vi "Get Device Type.vi"(8 "error in (no error)":errorcluster, 10 "config file refnum in":T2, 11 "IED in":refnum<class "IED.lvclass">) -> (0 "error out":errorcluster, 2 "config file refnum out":T2, 3 "IED out":refnum<class "IED.lvclass">, 4 "Device Type":T1)   [LabVIEW 2015, in "IED Actor.lvlib" / "IED.lvclass"]
uses:
  IED.lvclass
  <vilib>/Utility/config.llb/Config Data RefNum.ctl
  Controls/Device Type Enum.ctl
  <vilib>/Utility/config.llb/Read Key (String).vi
  <vilib>/Utility/config.llb/NI_LVConfig.lvlib
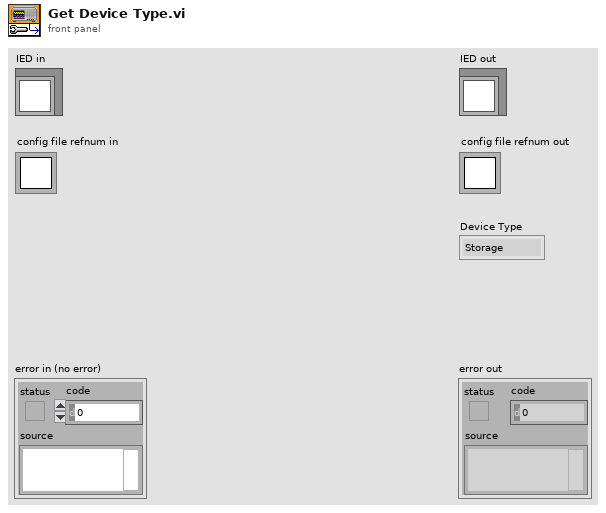
[diagram p1: front panel]
types:
  T1 = typedef "IED Actor.lvlib/IED.lvclass/Device Type Enum.ctl" = enum16{"Storage", "PV", "Generator", "Relay", "PCC", "Wind"}
  T2 = typedef "NI_LVConfig.lvlib/Config Data RefNum.ctl" = refnum<k1>
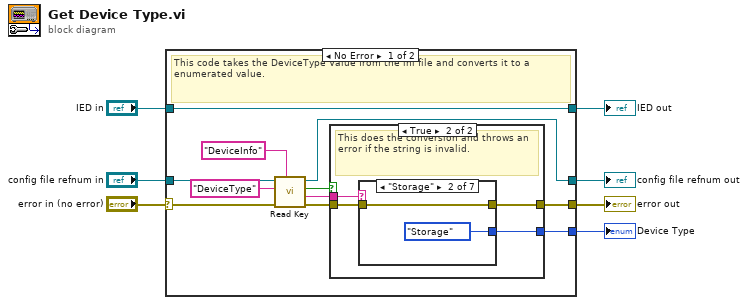
[diagram p0: block diagram]
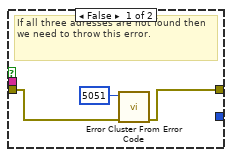
[diagram p2: hidden frame]
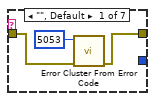
[diagram p3: hidden frame]
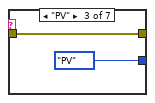
[diagram p4: hidden frame]
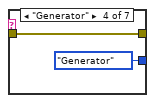
[diagram p5: hidden frame]
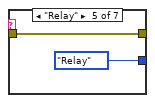
[diagram p6: hidden frame]
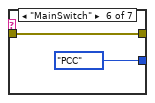
[diagram p7: hidden frame]
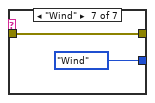
[diagram p8: hidden frame]
diagram:
  n1 = case shown="No Error" "error in (no error)" {
    selector: "error in (no error)" -> [w17 w43]
    tunnel: [w14 w43] -> w6
    tunnel: [w10 w42] -> w4
    tunnel: "IED in" -> [w10 w42]
    tunnel: "config file refnum in" -> [w18 w41]
    tunnel: [w8 w41] -> w2
    tunnel: [w9 _] -> w1
    frame No Error {
      # "This code takes the DeviceType Value from the ini file and converts it to a enumerated value."
      n2 = call-poly <vilib>:"Read Key.vi"("section"="DeviceInfo", "error in (no error)"=w17, "key"="DeviceType", "refnum"=w18) -> ("error out"=w12:errorcluster, "value"=w11:string, "found?"=w13:bool, "refnum out"=w8:T2)  [unwired: 4 in]
      n3 = case shown="True" w13 {
        tunnel: w12 -> [w21 w23]
        tunnel: [w19 w24] -> w14
        tunnel: w11 -> [_ w25]
        tunnel: [_ w22] -> w9
        frame False {
          # "If all three adresses are not found then we need to throw this error."
          n4 = call <vilib>:"Error Cluster From Error Code.vi"("error in (no error)"=w21, "error code (0)"=5051) -> ("error out"=w19:errorcluster)  [unwired: 7 in]
        }
        frame True {
          # "This does the conversion and throws an error if the string is invalid."
          n5 = case shown="\"Storage\"" w25 {
            tunnel: [w26 w30 w32 w34 w36 w38 w40] -> w24
            tunnel: w23 -> [w27 w30 w32 w34 w36 w38 w40]
            tunnel: [_ Device_Type_Enum."Storage" ("Device Type") Device_Type_Enum."PV" ("Device Type") Device_Type_Enum."Generator" ("Device Type") Device_Type_Enum."Relay" ("Device Type") Device_Type_Enum."PCC" ("Device Type") Device_Type_Enum."Wind" ("Device Type")] -> w22
            frame "", Default {
              n6 = call <vilib>:"Error Cluster From Error Code.vi"("error in (no error)"=w27, "error code (0)"=5053) -> ("error out"=w26:errorcluster)  [unwired: 7 in]
            }
            frame "Storage" {
            }
            frame "PV" {
            }
            frame "Generator" {
            }
            frame "Relay" {
            }
            frame "MainSwitch" {
            }
            frame "Wind" {
            }
          }
        }
      }
    }
    frame Error {
    }
  }
  "error out" <- w6
  "IED out" <- w4
  "config file refnum out" <- w2
  "Device Type" <- w1
